vi "Alice.vi"() -> ()   [LabVIEW 2013]
panel:
  out "error out 2":errorcluster
  out "error out":errorcluster
  in  "IP":string
  in  "Port":u16
  out "Ângulo Servo 2:":i32=90
  out "Bases escolhidas:":string="\n"
  out "Ângulo Servo 1:":i32
  out "Sinais enviados:":string
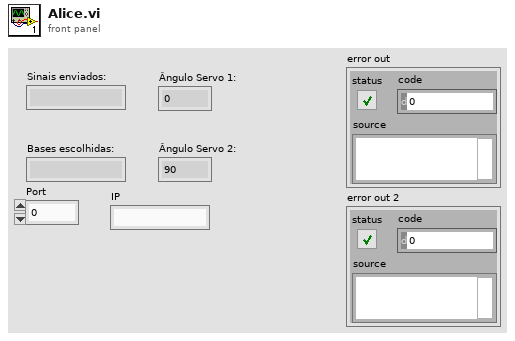
[diagram p1: front panel]
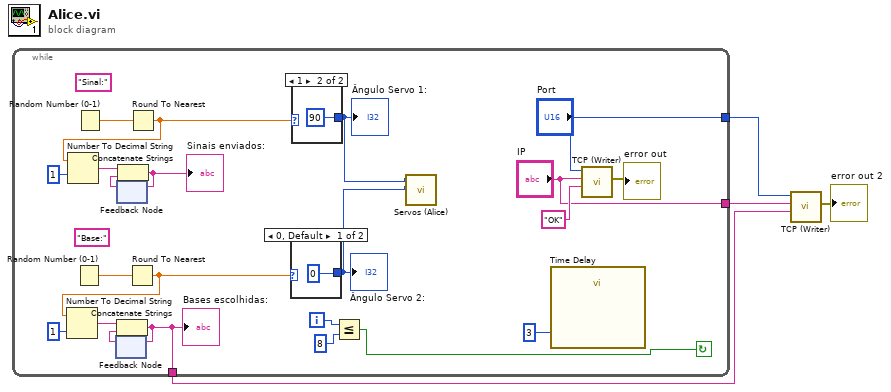
[diagram p0: block diagram]
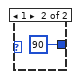
[diagram p2: hidden frame]
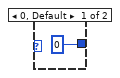
[diagram p3: hidden frame]
diagram:
  n1 = while {
    tunnel: ["Port"] -> w4
    tunnel: ["IP"] -> w3
    tunnel: [w5] -> w1
    i -> [w11]
    stop <- w14 continue-if-true
    (unwired) "Base:"
    (unwired) "Sinal:"
    n2 = Random Number (0-1)() -> (number: 0 to 1=w22:dbl)
    n3 = Random Number (0-1)() -> (number: 0 to 1=w26:dbl)
    n4 = feedback #1() -> (w20:string)  [unwired: 1 in]
    n5 = feedback #2() -> (w24:string)  [unwired: 1 in]
    n6 = Round To Nearest(number=w22) -> (nearest integer value=w19:dbl)
    n7 = Number To Decimal String(number=w19, width (-)=1) -> (decimal integer string=w21:string)
    n8 = Concatenate Strings(w21, w20) -> (w5:string)
    "Bases escolhidas:" <- w5
    n9 = feedback-in #1(w5) -> ()
    n10 = Round To Nearest(number=w26) -> (nearest integer value=w23:dbl)
    n11 = Number To Decimal String(number=w23, width (-)=1) -> (decimal integer string=w25:string)
    n12 = Concatenate Strings(w25, w24) -> (w6:string)
    "Sinais enviados:" <- w6
    n13 = feedback-in #2(w6) -> ()
    n14 = case shown="0, Default" w19 {
      tunnel: [0 90] -> w17
      frame 0, Default {
      }
      frame 1 {
      }
    }
    "Ângulo Servo 2:" <- w17
    n15 = case shown="1" w23 {
      tunnel: [0 90] -> w18
      frame 0, Default {
      }
      frame 1 {
      }
    }
    "Ângulo Servo 1:" <- w18
    n16 = Less Or Equal?(x=w11, y=8) -> (x <= y?=w14:bool)
    n17 = call "Servos (Alice).vi"("Servo 2:"=w17, "Servo 1:"=w18) -> ()  [unwired: 10 in]
    n18 = call "Time Delay"("Delay Time (s)"=3) -> ()  [unwired: 10 in, 1 out]
    n19 = call "TCP (Writer).vi"("data in"="OK", "IP"="IP", "Port"="Port") -> ("error out"=→"error out":errorcluster)  [unwired: 7 in, 1 out]
  }
  n20 = call "TCP (Writer).vi"("data in"=w1, "IP"=w3, "Port"=w4) -> ("error out"=→"error out 2":errorcluster)  [unwired: 7 in, 1 out]
